vi "BRig_dataLC_Wrong_OnOff_l1.vi"() -> (2 "output_Wrong_OnOff":i32)   [LabVIEW 2014]
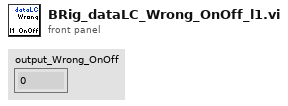
[diagram p1: front panel]
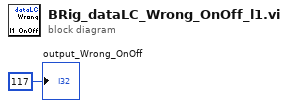
[diagram p0: block diagram]
diagram:
  "output_Wrong_OnOff" <- 117 ("output_iBlock")
